vi "getBounds.vi"(0 "reference":refnum<class "StateTransitionEdge.lvclass">, 1 "graphics":refnum<class "Graphics.lvclass">, 5 "error in (no error)":errorcluster) -> (14 "reference out":refnum<class "StateTransitionEdge.lvclass">, 15 "bounds":T1 {"height" format="%.2f"; "width" format="%.2f"; "y" format="%.2f"; "x" format="%.2f"}, 19 "error out":errorcluster)   [LabVIEW 2012, in "StateTransitionEdge.lvclass"]
doc: "public Rectangle2D getBounds(Graphics2D g2)"
uses:
  <resource>/Framework/Providers/Open_GDS/UML/StateTransitionEdge_class/StateTransitionEdge.lvclass
  <resource>/Framework/Providers/Open_GDS/UML/General/Rectangle/Rectangle Rectangle2D.ctl
  <resource>/Framework/Providers/Open_GDS/UML/Graphics_class/Graphics.lvclass
  <resource>/Framework/Providers/Open_GDS/UML/ClassRelationshipEdge_class/ClassRelationshipEdge.lvclass
  <resource>/Framework/Providers/Open_GDS/UML/SegmentedLineEdge_class/SegmentedLineEdge.lvclass
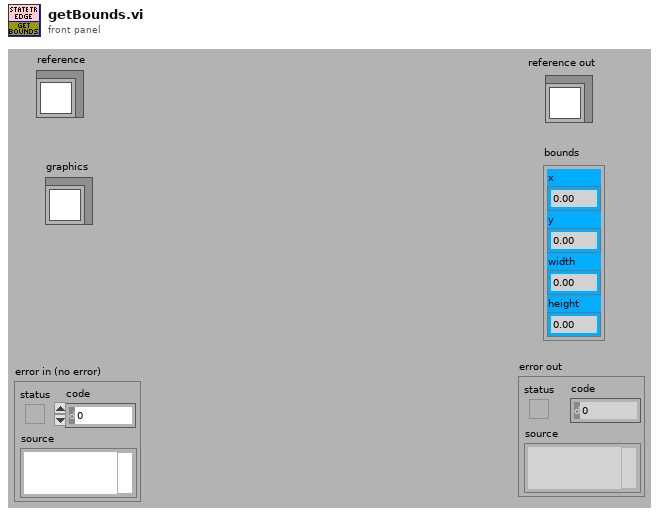
[diagram p1: front panel]
types:
  T1 = typedef "Rectangle Rectangle2D.ctl" = cluster{"x":dbl, "y":dbl, "width":dbl, "height":dbl}
  T2 = typedef "Point Point2D.ctl" = cluster{"x":dbl, "y":dbl}
  T3 = typedef "SegmentedLineEdge.lvclass/ObjectAttributes.ctl" = cluster{"lineStyle":refnum<class "LineStyle.lvclass">, "startArrowHead":refnum<class "ArrowHead.lvclass">, "endArrowHead":refnum<class "ArrowHead.lvclass">, "startLabel":string, "midLabel":string, "endLabel":string, "MidLabelOffset":T2, "SplitWire":bool}
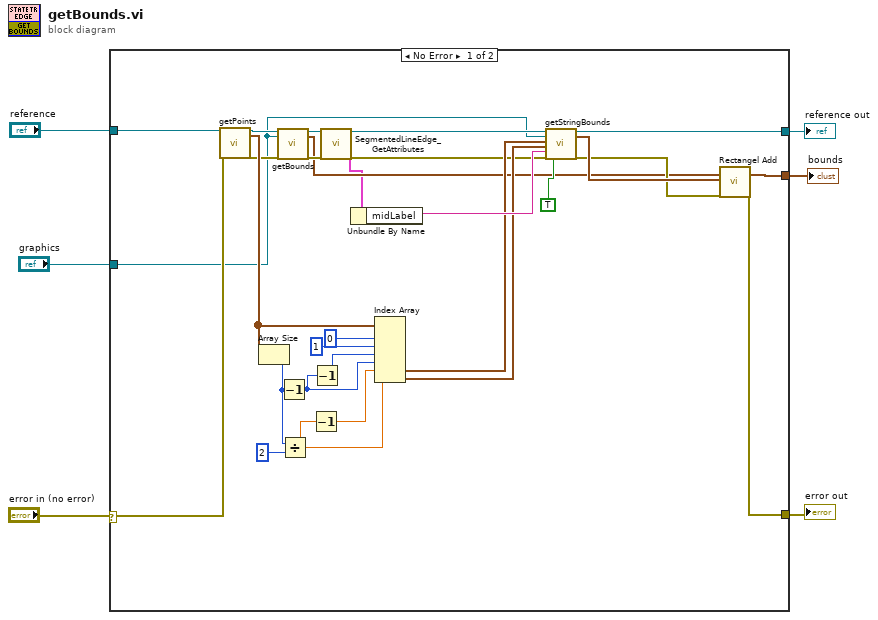
[diagram p0: block diagram]
diagram:
  n1 = case shown="No Error" "error in (no error)" {
    selector: "error in (no error)" -> [w19 w36]
    tunnel: "reference" -> [w35 w37]
    tunnel: [w34 w36] -> w5
    tunnel: [w14 w37] -> w4
    tunnel: "graphics" -> [w11 _]
    tunnel: [w33 _] -> w1
    frame No Error {
      n2 = call-dynamic "getPoints.vi"("reference"=w35, "error in (no error)"=w19) -> ("reference out"=w13:refnum<class "StateTransitionEdge.lvclass">, "points"=w29:T2[], "error out"=w12:errorcluster)  [unwired: 15 in]
      n3 = Array Size(array=w29) -> (size(s)=w25:i32)
      n4 = call-parent "getBounds.vi"("reference"=w13, "graphics"=w11, "error in (no error)"=w12) -> ("reference out"=w10:refnum<class "StateTransitionEdge.lvclass">, "bounds"=w8:T1, "error out"=w9:errorcluster)  [unwired: 14 in]
      n5 = Decrement(x=w25) -> (x-1=w28:i32)
      n6 = Divide(x=w25, y=2) -> (x/y=w24:dbl)
      n7 = Decrement(x=w24) -> (x-1=w23:dbl)
      n8 = Decrement(x=w28) -> (x-1=w27:i32)
      n9 = call <resource>:"SegmentedLineEdge_GetAttributes.vi"("reference in"=w10, "error in (no error)"=w9) -> ("reference out"=w15:refnum<class "StateTransitionEdge.lvclass">, "Data"=w7:T3, "error out"=w18:errorcluster)  [unwired: 14 in, 1 out]
      n10 = Unbundle By Name(w7) -> ("midLabel"=w32:string)
      n11 = Index Array(array=w29, index #1=0 ("index"), index #2=1 ("index"), index #3=w27, index #4=w28, index #5=w23, index #6=w24) -> (element #5=w22:T2, element #6=w21:T2)  [unwired: 4 out]
      n12 = call-dynamic "getStringBounds.vi"("reference"=w15, "graphics"=w11, "p1"=w22, "p2"=w21, "text"=w32, "error in (no error)"=w18, "center"=TRUE) -> ("reference out"=w14:refnum<class "StateTransitionEdge.lvclass">, "bounds"=w17:T1, "error out"=w16:errorcluster)  [unwired: 10 in]
      n13 = call <resource>:"Rectangel Add.vi"("bounds1"=w8, "bounds2"=w17, "error in (no error)"=w16) -> ("boundsAdded"=w33:T1, "error out"=w34:errorcluster)  [unwired: 2 in, 13 out]
    }
    frame Error {
    }
  }
  "reference out" <- w4
  "error out" <- w5
  "bounds" <- w1
